vi "ADC_get_point.vi"(2 "Readout parameter":T1, 3 "Integration time (ms)":u32) -> (0 "data":dbl[](array[numeric]))   [LabVIEW 2013]
uses:
  <vilib>/DAQmx/read.llb/DAQmx Read (Analog 2D DBL NChan NSamp).vi
  <vilib>/Analysis/baseanly.llb/A x Vector.vi
  <vilib>/DAQmx/miscellaneous.llb/DAQmx Fill In Error Info.vi
  <vilib>/Analysis/NI_AALBase.lvlib
  <resource>/objmgr/daqmx.rc
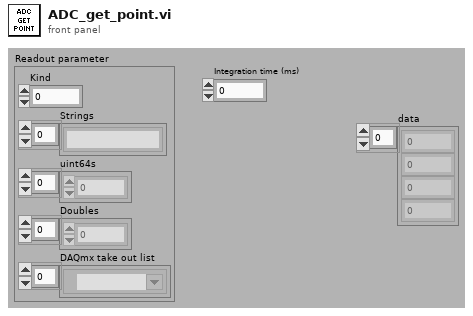
[diagram p1: front panel]
types:
  T1 = cluster{"Kind":u16, "Strings":string[], "uint64s":u64[], "Doubles":dbl[], "DAQmx take out list":refnum<k21>[]}
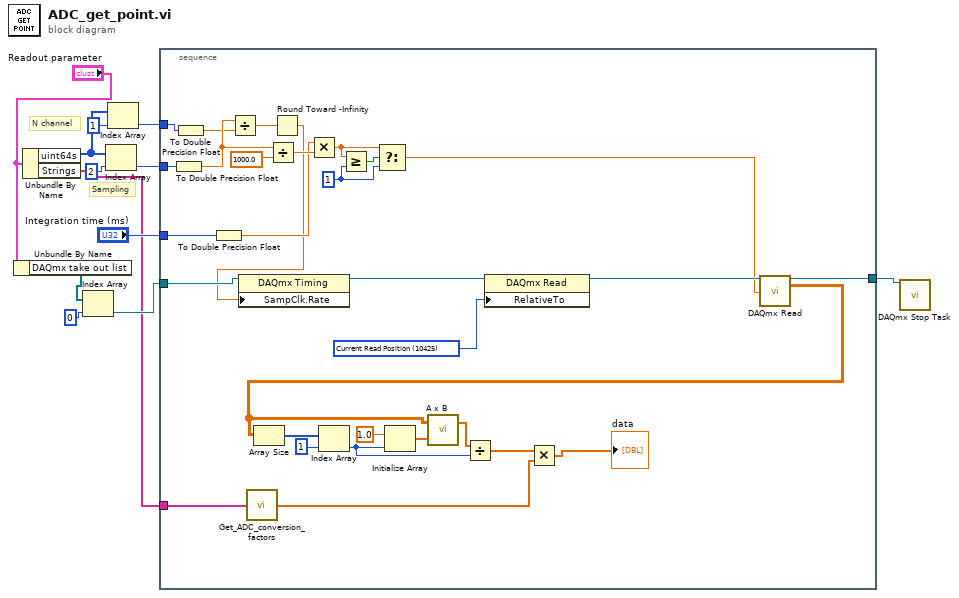
[diagram p0: block diagram]
diagram:
  # "Sampling"
  # "N channel"
  n1 = Unbundle By Name("Readout parameter") -> ("DAQmx take out list"=w4:refnum<k21>[])
  n2 = Unbundle By Name("Readout parameter") -> ("uint64s"=w12:u64[], "Strings"=w1:string[])
  n3 = Index Array(array=w4, index=0) -> (element=w2:refnum<k21>)
  n4 = Index Array(array=w12, index=2) -> (element=w9:u64)
  n5 = Index Array(array=w12, index=1) -> (element=w8:u64)
  n6 = stacked-sequence {
    tunnel: w9 -> [w35]
    tunnel: w8 -> [w36]
    tunnel: "Integration time (ms)" -> [w34]
    tunnel: w2 -> [w27]
    tunnel: [w17] -> w6
    tunnel: w1 -> [w16]
    frame #0 {
      w28 = 10425 items=["First Sample"=10424, "Current Read Position"=10425, "Reference Trigger"=10426, "First Pretrigger Sample"=10427, "Most Recent Sample"=10428] ("RelativeTo")
      w41 = 1 ("y")
      n7 = To Double Precision Float(number=w35) -> (double precision float=w32:dbl)
      n8 = To Double Precision Float(number=w36) -> (double precision float=w31:dbl)
      n9 = To Double Precision Float(number=w34) -> (double precision float=w33:dbl)
      n10 = Divide(x=w32, y=w31) -> (x/y=w39:dbl)
      n11 = call "Get_ADC_conversion_factors.vi"("Strings"=w16) -> ("Conversion factors"=w14:dbl[])
      n12 = Divide(x=w32, y=1000.0) -> (x/y=w38:dbl)
      n13 = Round Toward -Infinity(1:w39) -> (0:w26:dbl)
      n14 = property class="DAQmx Timing"(reference=w27, "SampClk.Rate"=w26) -> (reference out=w30:refnum<k21>)  [unwired: 1 in, 1 out]
      n15 = Multiply(x=w33, y=w38) -> (x*y=w37:dbl)
      n16 = Greater Or Equal?(x=w37, y=w41) -> (x >= y?=w42:bool)
      n17 = Select(t=w37, s=w42, f=w41) -> (s? t:f=w25:dbl)
      n18 = property class="DAQmx Read"(reference=w30, "RelativeTo"=w28) -> (reference out=w29:refnum<k21>)  [unwired: 1 in, 1 out]
      n19 = call-poly <vilib>:"DAQmx Read.vi"("task/channels in"=w29, "number of samples per channel"=w25) -> ("task out"=w17:refnum<k21>, "data"=w18:dbl[][])  [unwired: 11 in, 1 out]
      n20 = Array Size(array=w18) -> (size(s)=w22:i32[])
      n21 = Index Array(array=w22, index=1) -> (element=w19:i32)
      n22 = Initialize Array(1.0 ("element"), w19) -> (w23:dbl[])
      n23 = call-poly <vilib>:"A x B.vi"("Vector"=w23, "A"=w18) -> ("A x Vector"=w20:dbl[])  [unwired: 1 out]
      n24 = Divide(x=w20, y=w19) -> (x/y=w15:dbl[])
      n25 = Multiply(x=w15, y=w14) -> (x*y=→"data":dbl[])
    }
  }
  n26 = call <vilib>:"DAQmx Stop Task.vi"("task/channels in"=w6) -> ()  [unwired: 13 in, 2 out]
